vi "_blacklist.vi"() -> (3 "blacklist":string[](array[string]))   [LabVIEW 2014, in "RefManager(dev).lvlib"]
uses:
  RefManager(dev).lvlib
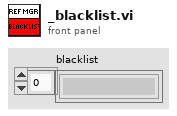
[diagram p1: front panel]
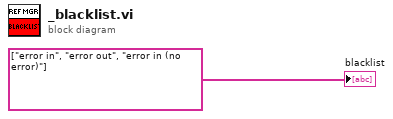
[diagram p0: block diagram]
diagram:
  "blacklist" <- string[] ["error in", "error out", "error in (no error)"] ("blacklist")
